vi "Send Configure Power Line Frequency [PLF].vi"(7 "Message Priority (Normal)":T1=enum."Normal", 8 "error in (no error)":errorcluster, 10 "power line frequency (60.0 Hz)":dbl=60.0 format="%^.2e", 11 "Message Enqueuer":refnum<class "Message Enqueuer.lvclass">) -> (0 "error out":errorcluster, 3 "Message Enqueuer out":refnum<class "Message Enqueuer.lvclass">)   [LabVIEW 2015, in "CS++DMM.lvlib" / "Configure Power Line Frequency [PLF] Msg.lvclass"]
doc: "Sends the <B>CS++DMM.lvlib:Configure Power Line Frequency [PLF] Msg.lvclass</B> message.\n\n<B>CS++DMM.lvlib:CS++DMM.lvclass:Configure Power Line Frequency [PLF].vi</B> Description:\n\nThis VI configures the power line frequency of the DMM.\n\nNote:\n\n(1) This VI is part of the IviDmmPowerLineFrequency [PLF] extension group."
uses:
  Configure Power Line Frequency [PLF] Msg.lvclass
  <vilib>/ActorFramework/Message Enqueuer/Message Enqueuer.lvclass
  <vilib>/ActorFramework/Message Enqueuer/Message Priority.ctl
  Configure Power Line Frequency [PLF] Msg.lvclass/Configure Power Line Frequency [PLF] Msg.ctl
  <vilib>/ActorFramework/Message Enqueuer/Message Enqueuer.lvclass/Message Enqueuer.ctl
  <vilib>/ActorFramework/Message Priority Queue/Priority Enqueue.vi
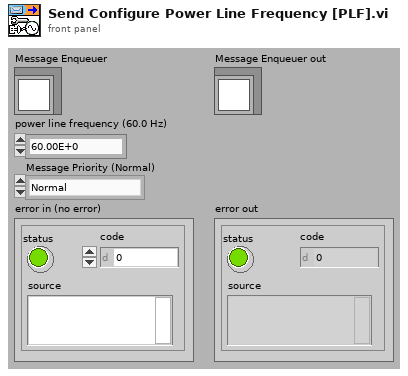
[diagram p1: front panel]
types:
  T1 = typedef "Actor Framework.lvlib/Message Enqueuer.lvclass/Message Priority.ctl" = enum16{"Low", "Normal", "High"}
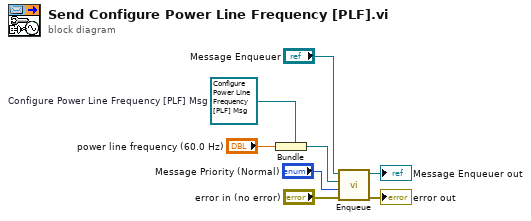
[diagram p0: block diagram]
diagram:
  w2 = refnum<class "Configure Power Line Frequency [PLF] Msg.lvclass"> refnum  # Configure Power Line Frequency [PLF] Msg
  n1 = Bundle(cluster=w2, "power line frequency (60.0 Hz)") -> (w5:refnum<class "Configure Power Line Frequency [PLF] Msg.lvclass">)
  n2 = call <vilib>:"Enqueue.vi"("error in (no error)"="error in (no error)", "Message Priority (Normal)"="Message Priority (Normal)", "Message"=w5, "Message Enqueuer in"="Message Enqueuer") -> ("error out"=→"error out":errorcluster, "Message Enqueuer out"=→"Message Enqueuer out":refnum<class "Message Enqueuer.lvclass">)  [unwired: 6 in]
